vi "TempHumWindDir_Calibration.vi"() -> ()   [LabVIEW 2012]
panel:
  out "Wind dir.":i32
  out "Hum. in":dbl
  out "Hum. out":dbl
  out "Temp. out":dbl
  out "Temp. in":dbl
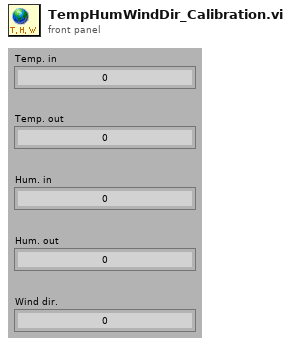
[diagram p1: front panel]
diagram:
